vi "Translator.SelectLanguageGui.vi"() -> (1 "english":bool, 2 "changed":bool, 3 "Language":string)   [LabVIEW 2016]
uses:
  Translator.SelectLanguageGui.Action.ctl
  <vilib>/Utility/miscctls.llb/LVBoundsTypeDef.ctl
  Translator.Global.vi
  Config/Config.Global.vi
panel:
  out "init val":u16
  out "_loop":i32(ring)=4
  in  "_Language":u16(ring) caption="Select Language..." items=["English"]
  in  "CancelButton":bool
  in  "OKButton":bool
  out "~flag":picture
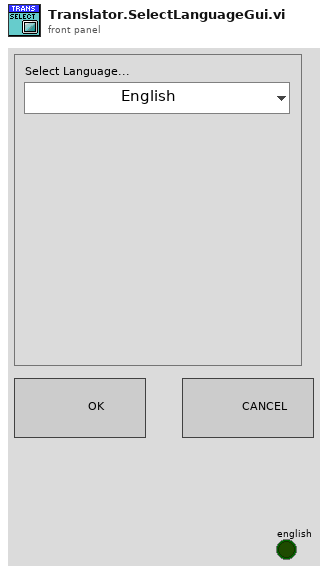
[diagram p1: front panel]
types:
  T1 = typedef "Translator.SelectLanguageGui.Action.ctl" = enum32{"idle", "constructor", "destructor", "--- SelectLang ---"}
  T2 = enum32{"invalid app kind", "Development System", "Run Time System", "Student Edition", "Embedded LabVIEW", "Evaluation", "Custom"}
  T3 = typedef "LVBoundsTypeDef.ctl" = cluster{"Width":u32, "Height":u32}
  T4 = typedef "LVPositionTypeDef.ctl" = cluster{"Left":i32, "Top":i32}
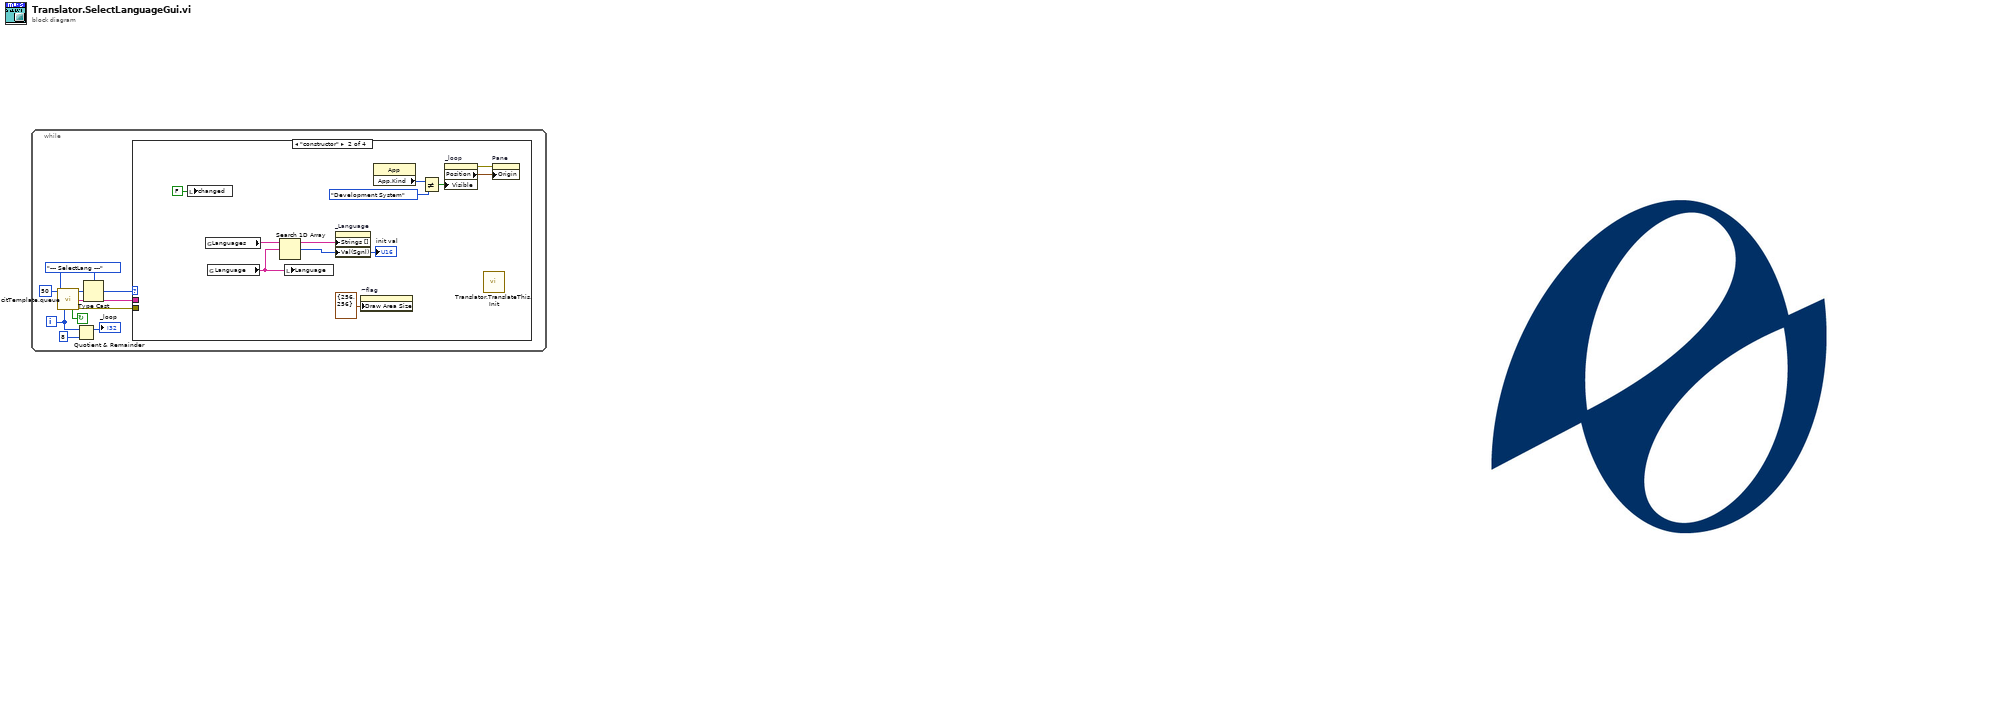
[diagram p0: block diagram]
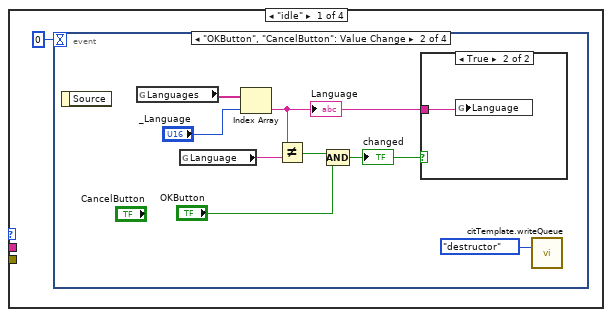
[diagram p2: hidden frame]
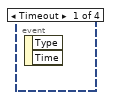
[diagram p3: hidden frame]
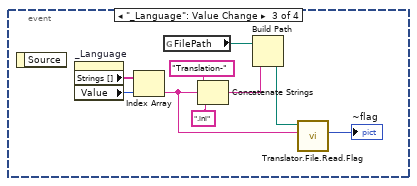
[diagram p5: hidden frame]
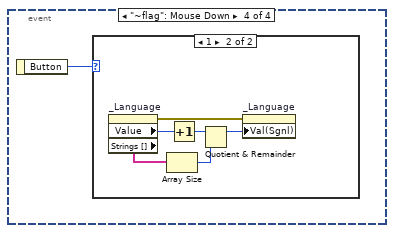
[diagram p6: hidden frame]
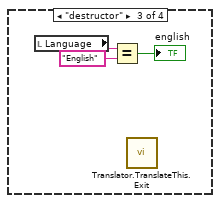
[diagram p8: hidden frame]
diagram:
  n1 = while {
    i -> [w1]
    stop <- w10 continue-if-true
    w4 = Translator.SelectLanguageGui.Action."--- SelectLang ---" ("Action")
    n2 = call "citTemplate.queue.vi"("ms timeout (250 ms)"=50, "event enum"=w4, "iteration (-1)"=w1) -> ("event out"=w8:u32, "(flatten) data out"=w5:string, "continue"=w10:bool, "error out"=w6:errorcluster)  [unwired: 2 in, 7 out]
    n3 = Quotient & Remainder(x=w1, y=8) -> (x-y*floor(x/y)=→"_loop":i32)  [unwired: 1 out]
    n4 = Type Cast(type=w4, x=w8) -> (*(type *) &x=w7:T1)
    n5 = case shown="\"constructor\"" w7 {
      tunnel: w6 -> [_ _ _ _]
      tunnel: w5 -> [_ _ _ _]
      frame "idle" {
        n6 = event shown="[1] \"OKButton\", \"CancelButton\": Value Change" {
          selector: _ -> [_ _ _ _]
          dyn-events: _ -> [_ _ _ _]
          timeout: 0 -> [_ _ _ _]
          event Timeout {
            n7 = event-data() -> ()  [unwired: 3 out]
          }
          event "OKButton", "CancelButton": Value Change {
            n8 = event-data() -> ()  [unwired: 2 out]
            n9 = global read "Translator.Global.vi" "Languages"() -> (w17:string[])
            n10 = global read "Config.Global.vi" "Language"() -> (w15:string)
            n11 = Index Array(array=w17, index="_Language") -> (element=w12:string)
            "Language" <- w12
            n12 = Not Equal?(x=w12, y=w15) -> (x != y?=w19:bool)
            n13 = Compound Arithmetic op=AND(w19, "OKButton") -> (w13:bool)
            "changed" <- w13
            n14 = case shown="True" w13 {
              tunnel: w12 -> [_ w20]
              frame False {
              }
              frame True {
                n15 = global write "Config.Global.vi" "Language"(w20) -> ()
              }
            }
            n16 = call "citTemplate.writeQueue.vi"("event in (if not connected:all statemachine with data event)"=Translator.SelectLanguageGui.Action."destructor" ("Action")) -> ()  [unwired: 14 in, 1 out]
          }
          event "_Language": Value Change {
            n17 = event-data() -> ()  [unwired: 2 out]
            n18 = property on="_Language" class="Ring (strict)"() -> ("Strings []"=w27:string[], "Value"=w28:u16)  [unwired: 2 in, 2 out]
            n19 = Index Array(array=w27, index=w28) -> (element=w23:string)
            n20 = global read "Translator.Global.vi" "FilePath"() -> (w21:path)
            n21 = Concatenate Strings("Translation-" ("string"), w23, ".ini" ("string")) -> (w26:string)
            n22 = Build Path(base path=w21, name or relative path=w26) -> (appended path=w29:path)
            n23 = call "Translator.File.Read.Flag.vi"("Language in use"=w23, "Translation file"=w29) -> ("~flag"=→"~flag":picture)  [unwired: 7 in, 2 out]
          }
          event "~flag": Mouse Down {
            n24 = event-data() -> ("Button"=w30:u16)  [unwired: 1 out]
            n25 = case shown="1" w30 {
              frame 0, Default {
              }
              frame 1 {
                n26 = property on="_Language" class="Ring (strict)"() -> (error out=w36:errorcluster, "Value"=w35:u16, "Strings []"=w31:string[])  [unwired: 2 in, 1 out]
                n27 = Array Size(array=w31) -> (size(s)=w32:i32)
                n28 = Increment(x=w35) -> (x+1=w34:u16)
                n29 = Quotient & Remainder(x=w34, y=w32) -> (x-y*floor(x/y)=w33:i32)  [unwired: 1 out]
                n30 = property on="_Language" class="Ring (strict)"(error in=w36, "Val(Sgnl)"=w33) -> ()  [unwired: 1 in, 2 out]
              }
            }
          }
        }
      }
      frame "constructor" {
        n31 = local write "changed"(FALSE ("_b_ok")) -> ()
        n32 = global read "Translator.Global.vi" "Languages"() -> (w44:string[])
        n33 = global read "Config.Global.vi" "Language"() -> (w43:string)
        n34 = Search 1D Array(1D array=w44, element=w43) -> (index of element=w37:i32)  [unwired: 1 in]
        "init val" <- w37
        n35 = local write "Language"(w43) -> ()
        n36 = property on="_Language" class="Ring (strict)"("Strings []"=w44, "Val(Sgnl)"=w37) -> ()  [unwired: 2 in, 2 out]
        n37 = property on="~flag" class="Pict"("Draw Area Size"=T3 {"Width"=256, "Height"=256}) -> ()  [unwired: 2 in, 2 out]
        n38 = property class="App"() -> ("App.Kind"=w40:T2)  [unwired: 2 in, 2 out]
        n39 = Not Equal?(x=w40, y=T2."Development System") -> (x != y?=w38:bool)
        n40 = property on="_loop" class="Ring (strict)"("Visible"=w38) -> (error out=w42:errorcluster, "Position"=w41:T4)  [unwired: 2 in, 1 out]
        n41 = call "Translator.TranslateThis.Init.vi"() -> ()  [unwired: 11 in, 1 out]
        n42 = property on="Pane" class="Pane"(error in=w42, "Origin"=w41) -> ()  [unwired: 1 in, 2 out]
      }
      frame "destructor" {
        n43 = local read "Language"() -> (w47:string)
        n44 = Equal?(x=w47, y="English") -> (x = y?=→"english":bool)
        n45 = call "Translator.TranslateThis.Exit.vi"() -> ()  [unwired: 11 in, 1 out]
      }
      frame "--- SelectLang ---" {
      }
    }
  }
